vi "SD Write Boolean Rarely.vi"(8 "Iteration":i32=10, 9 "Boolean":bool, 11 "Name":string="Numeric") -> ()   [LabVIEW 2013]
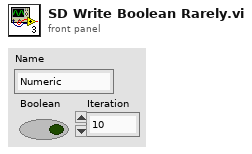
[diagram p1: front panel]
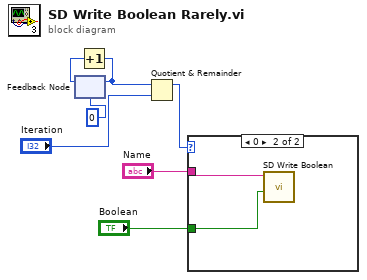
[diagram p0: block diagram]
diagram:
  n1 = feedback #1(0) -> (w5:i32)
  n2 = Increment(x=w5) -> (x+1=w4:i32)
  n3 = feedback-in #1(w4) -> ()
  n4 = Quotient & Remainder(x=w4, y="Iteration") -> (x-y*floor(x/y)=w2:i32)  [unwired: 1 out]
  n5 = case shown="0" w2 {
    tunnel: "Name" -> [_ w9]
    tunnel: "Boolean" -> [_ w8]
    frame Default {
    }
    frame 0 {
      n6 = call <vilib>:"SD Write Boolean.vi"("Boolean"=w8, "Name"=w9) -> ()  [unwired: 8 in, 2 out]
    }
  }
